vi "Autonomia SUB1  v1.vi"(11 "Ster Wej":cluster{dbl, dbl}) -> (1 "wyj pred":cluster{u16, u16, u16, u16, u16, u16} {"?" scale=0.0..65000.0; "?" scale=0.0..65000.0; "?" scale=0.0..65000.0; "?" scale=0.0..65000.0; "?" scale=0.0..65000.0; "?" scale=0.0..65000.0}, 2 "P 6":dbl(slide) scale=-66000.0..66000.0, 3 "P 7":dbl(slide) scale=-66000.0..66000.0, 4 "L 7":dbl(slide) scale=-66000.0..66000.0, 5 "P 5":dbl(slide) scale=-66000.0..66000.0, 6 "L 6":dbl(slide) scale=-66000.0..66000.0, 7 "L 5":dbl(slide) scale=-66000.0..66000.0)   [LabVIEW 2014]
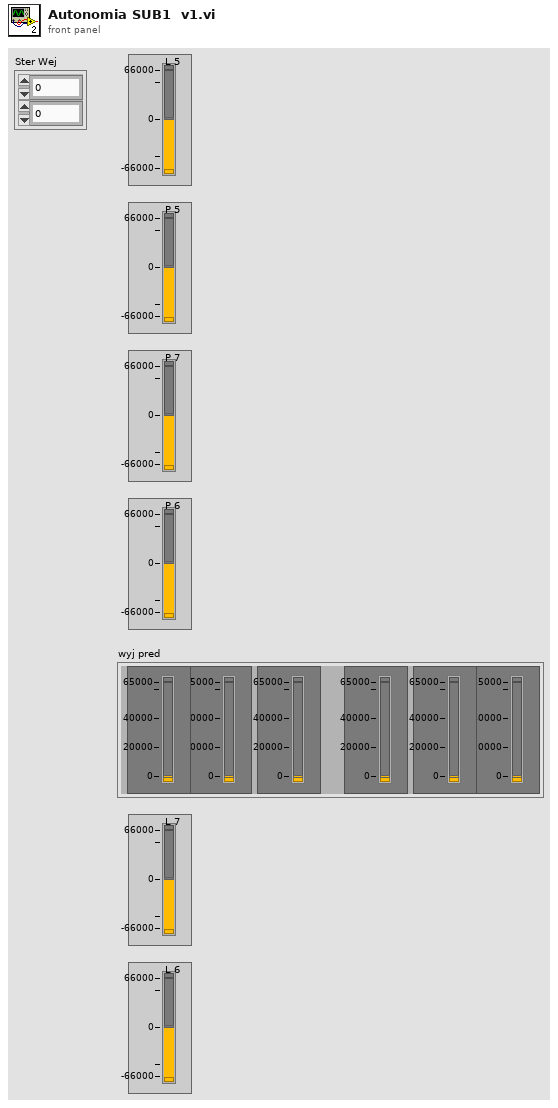
[diagram p1: front panel]
types:
  T1 = cluster{"p1":dbl, "p2":dbl, "p3":dbl, "l1":dbl, "l2":dbl, "l3":dbl}
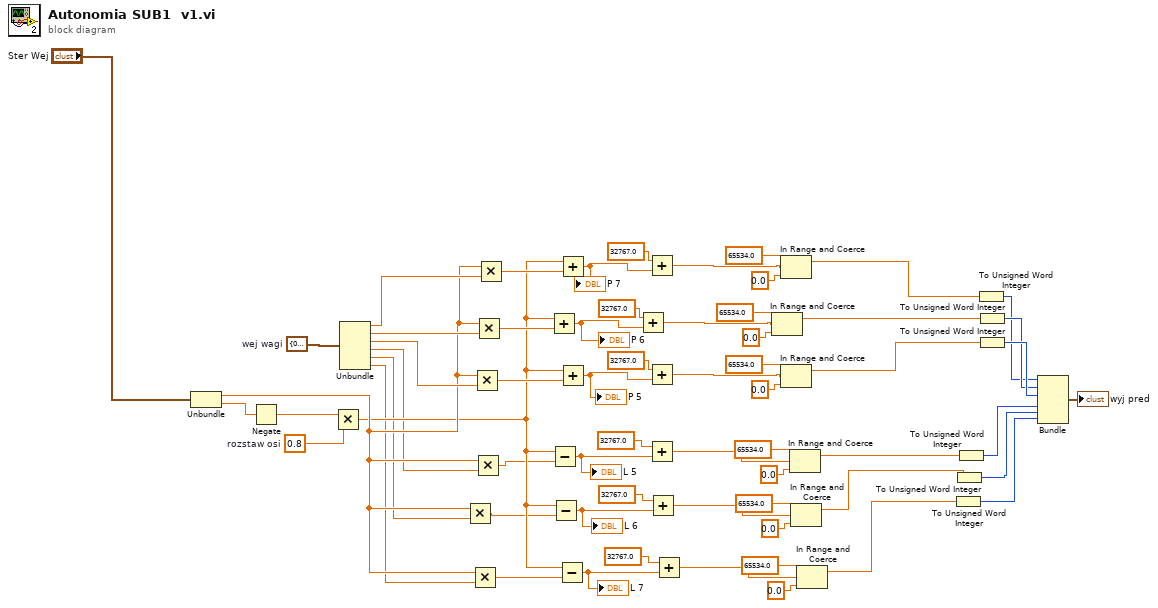
[diagram p0: block diagram]
diagram:
  w61 = T1 {"p1"=0.0, "p2"=0.0, "p3"=0.0, "l1"=0.0, "l2"=0.0, "l3"=0.0}  # wej wagi
  w6 = 0.8  # rozstaw osi
  n1 = Unbundle("Ster Wej") -> (w54:dbl, w7:dbl)
  n2 = Negate(x=w7) -> (-x=w15:dbl)
  n3 = Multiply(x=w15, y=w6) -> (x*y=w53:dbl)
  n4 = Unbundle(w61) -> ("p1"=w55:dbl, "p2"=w56:dbl, "p3"=w57:dbl, "l1"=w37:dbl, "l2"=w38:dbl, "l3"=w39:dbl)
  n5 = Multiply(x=w54, y=w38) -> (x*y=w32:dbl)
  n6 = Multiply(x=w54, y=w39) -> (x*y=w33:dbl)
  n7 = Multiply(x=w54, y=w57) -> (x*y=w60:dbl)
  n8 = Multiply(x=w54, y=w37) -> (x*y=w31:dbl)
  n9 = Multiply(x=w54, y=w56) -> (x*y=w59:dbl)
  n10 = Multiply(x=w54, y=w55) -> (x*y=w58:dbl)
  n11 = Add(x=w53, y=w59) -> (x+y=w41:dbl)
  "P 6" <- w41
  n12 = Subtract(x=w53, y=w31) -> (x-y=w17:dbl)
  "L 5" <- w17
  n13 = Subtract(x=w53, y=w32) -> (x-y=w23:dbl)
  "L 6" <- w23
  n14 = Subtract(x=w53, y=w33) -> (x-y=w28:dbl)
  "L 7" <- w28
  n15 = Add(x=w53, y=w58) -> (x+y=w48:dbl)
  "P 7" <- w48
  n16 = Add(x=w53, y=w60) -> (x+y=w16:dbl)
  "P 5" <- w16
  n17 = Add(x=32767.0 ("y"), y=w41) -> (x+y=w40:dbl)
  n18 = Add(x=32767.0 ("y"), y=w48) -> (x+y=w49:dbl)
  n19 = Add(x=32767.0 ("y"), y=w16) -> (x+y=w19:dbl)
  n20 = Add(x=32767.0 ("y"), y=w17) -> (x+y=w18:dbl)
  n21 = Add(x=32767.0 ("y"), y=w23) -> (x+y=w22:dbl)
  n22 = Add(x=32767.0 ("y"), y=w28) -> (x+y=w29:dbl)
  n23 = In Range and Coerce(upper limit=65534.0 ("y"), x=w40, lower limit=0.0 ("y")) -> (coerced(x)=w51:dbl)  [unwired: 1 out]
  n24 = In Range and Coerce(upper limit=65534.0 ("y"), x=w49, lower limit=0.0 ("y")) -> (coerced(x)=w52:dbl)  [unwired: 1 out]
  n25 = In Range and Coerce(upper limit=65534.0 ("y"), x=w19, lower limit=0.0 ("y")) -> (coerced(x)=w50:dbl)  [unwired: 1 out]
  n26 = In Range and Coerce(upper limit=65534.0 ("y"), x=w18, lower limit=0.0 ("y")) -> (coerced(x)=w34:dbl)  [unwired: 1 out]
  n27 = In Range and Coerce(upper limit=65534.0 ("y"), x=w22, lower limit=0.0 ("y")) -> (coerced(x)=w35:dbl)  [unwired: 1 out]
  n28 = In Range and Coerce(upper limit=65534.0 ("y"), x=w29, lower limit=0.0 ("y")) -> (coerced(x)=w36:dbl)  [unwired: 1 out]
  n29 = To Unsigned Word Integer(number=w36) -> (unsigned 16bit integer=w13:u16)
  n30 = To Unsigned Word Integer(number=w35) -> (unsigned 16bit integer=w12:u16)
  n31 = To Unsigned Word Integer(number=w34) -> (unsigned 16bit integer=w11:u16)
  n32 = To Unsigned Word Integer(number=w52) -> (unsigned 16bit integer=w8:u16)
  n33 = To Unsigned Word Integer(number=w51) -> (unsigned 16bit integer=w9:u16)
  n34 = To Unsigned Word Integer(number=w50) -> (unsigned 16bit integer=w10:u16)
  n35 = Bundle(w8, w9, w10, w11, w12, w13) -> (→"wyj pred":cluster{u16, u16, u16, u16, u16, u16})  [unwired: 1 in]
